vi "Experiment03.vi"() -> ()   [LabVIEW 2009]
uses:
  <vilib>/imath/engines/lvmath2/RunTimeEngine/ErrorHandling/NIMS_Finalize Error.vi
  <vilib>/imath/engines/lvmath2/RunTimeEngine/Parser/MC_Version.vi
  <vilib>/imath/engines/lvmath2/RunTimeEngine/Managers/WorkSpace/UID Generator.vi
  <vilib>/imath/engines/lvmath/Functions/Error Handling/error.ctl
  <vilib>/imath/engines/lvmath2/RunTimeEngine/NodeEndStatement/NIMS_NodeEndStatement_Output.vi
  <instcachedir>/0/NIMS_NodeEndStatement_Output_B70DDD75627E4997AAE11E9955EDAA25.lvgen/NIMS_NodeEndStatement_Output_B70DDD75627E4997AAE11E9955EDAA25_000.vi
  <vilib>/imath/engines/lvmath2/RunTimeEngine/Managers/SymbolTable/Clear UID.vi
  <vilib>/imath/engines/lvmath/Functions/Error Handling/MergeErrorsWrapper.vi
  <vilib>/imath/engines/lvmath2/RunTimeEngine/VariableToken/NIMS_VariableToken_CondDefined.vi
  <instcachedir>/0/NIMS_VariableToken_CondDefined_5641E79000FB4D628475532441475385.lvgen/NIMS_VariableToken_CondDefined_5641E79000FB4D628475532441475385_001.vi
  <vilib>/imath/engines/lvmath/Functions/Error Handling/MC_Mask_Errors.vi
  <vilib>/imath/engines/lvmath2/RunTimeEngine/BuiltInFunctions/rem/NIMS_rem_no checks.vi
  <instcachedir>/0/NIMS_rem_no checks_4CC9B305AB7E42EF90AFC4973FB32F8D.lvgen/NIMS_rem_no checks_4CC9B305AB7E42EF90AFC4973FB32F8D_000.vi
  <vilib>/imath/engines/lvmath2/RunTimeEngine/BuiltInFunctions/uint32/NIMS_uint32(real).vi
  <instcachedir>/0/NIMS_uint32(real)_FDC83D68D45943DDB8F3F934FF8A712F.lvgen/NIMS_uint32(real)_FDC83D68D45943DDB8F3F934FF8A712F_000.vi
  <vilib>/imath/engines/lvmath2/RunTimeEngine/BuiltInFunctions/double/NIMS_double.vi
  <instcachedir>/0/NIMS_double_2CE444F3CE4146B199A482FE12545E45.lvgen/NIMS_double_2CE444F3CE4146B199A482FE12545E45_000.vi
  <vilib>/imath/engines/lvmath2/RunTimeEngine/RangeToken/NIMS_Range.vi
  <instcachedir>/0/NIMS_Range_6D647EC16A744C98B5DE1D649A2D648D.lvgen/NIMS_Range_6D647EC16A744C98B5DE1D649A2D648D_001.vi
  <vilib>/imath/engines/lvmath2/RunTimeEngine/BuiltInFunctions/length/NIMS_length(GV).vi
  <instcachedir>/0/NIMS_length(GV)_7D6E94E728E145E68721C53861296D96.lvgen/NIMS_length(GV)_7D6E94E728E145E68721C53861296D96_000.vi
  <instcachedir>/0/NIMS_Range_6D647EC16A744C98B5DE1D649A2D648D.lvgen/NIMS_Range_6D647EC16A744C98B5DE1D649A2D648D_000.vi
  <vilib>/imathl/engines/lvmath/Functions/Error Handling/Create Error.vi
  <vilib>/imath/engines/lvmath2/RunTimeEngine/ReplaceToken/NIMS_Replace - V(S)=S.vi
  <instcachedir>/0/NIMS_Replace - V(S)=S_670A9E0533664C1D848C8E58B3321B6A.lvgen/NIMS_Replace - V(S)=S_670A9E0533664C1D848C8E58B3321B6A_002.vi
  <vilib>/imath/engines/lvmath2/RunTimeEngine/ReplaceToken/NIMS_Replace - Size Check _(_)=S.vi
  <instcachedir>/0/NIMS_Replace - Size Check _(_)=S_8596181D73404097BAB9CBB006194BB0.lvgen/NIMS_Replace - Size Check _(_)=S_8596181D73404097BAB9CBB006194BB0_002.vi
  <vilib>/imath/engines/lvmath2/RunTimeEngine/ReplaceToken/NIMS_Replace - Check Linear.vi
  <instcachedir>/0/NIMS_Replace - Check Linear_9243CBB174894FF6977027453DA6955E.lvgen/NIMS_Replace - Check Linear_9243CBB174894FF6977027453DA6955E_002.vi
  <vilib>/imath/engines/lvmath2/RunTimeEngine/VariableToken/NIMS_VariableToken_CondDefinedDefinedByReplace.vi
  <instcachedir>/0/NIMS_VariableToken_CondDefinedDefinedByReplace_D162CFFC24174562A9FEA619A91E1A56.lvgen/NIMS_VariableToken_CondDefinedDefinedByReplace_D162CFFC24174562A9FEA619A91E1A56_002.vi
  <vilib>/imath/engines/lvmath2/RunTimeEngine/CommandStatement/MC_CommandStatement_break.vi
  <vilib>/imath/engines/lvmath2/RunTimeEngine/LocalVariableDefStatement/MC_LocalVariableDefStatement_Display.vi
  <vilib>/imath/engines/lvmath2/RunTimeEngine/RunTimeType/NIMS_RunTimeType_From StrictType (excl LVString).vi
  <vilib>/imath/engines/lvmath2/RunTimeEngine/ArithmeticOperatorToken/NIMS_ArithmeticOperator_times.vi
  <instcachedir>/0/NIMS_ArithmeticOperator_times_3987BC660D7947CD8628C10658A43225.lvgen/NIMS_ArithmeticOperator_times_3987BC660D7947CD8628C10658A43225_001.vi
  <instcachedir>/0/NIMS_NodeEndStatement_Output_B70DDD75627E4997AAE11E9955EDAA25.lvgen/NIMS_NodeEndStatement_Output_B70DDD75627E4997AAE11E9955EDAA25_001.vi
  <instcachedir>/0/NIMS_ArithmeticOperator_times_3987BC660D7947CD8628C10658A43225.lvgen/NIMS_ArithmeticOperator_times_3987BC660D7947CD8628C10658A43225_000.vi
  <vilib>/imath/engines/lvmath2/RunTimeEngine/VariableToken/Read/NIMS_Get Elements - RV(_) - Check.vi
  <instcachedir>/0/NIMS_Get Elements - RV(_) - Check_60F12861D0564803969A5D0D0D1716CD.lvgen/NIMS_Get Elements - RV(_) - Check_60F12861D0564803969A5D0D0D1716CD_000.vi
  <instcachedir>/0/NIMS_NodeEndStatement_Output_B70DDD75627E4997AAE11E9955EDAA25.lvgen/NIMS_NodeEndStatement_Output_B70DDD75627E4997AAE11E9955EDAA25_003.vi
  <instcachedir>/0/NIMS_VariableToken_CondDefined_5641E79000FB4D628475532441475385.lvgen/NIMS_VariableToken_CondDefined_5641E79000FB4D628475532441475385_000.vi
  <instcachedir>/0/NIMS_Replace - V(S)=S_670A9E0533664C1D848C8E58B3321B6A.lvgen/NIMS_Replace - V(S)=S_670A9E0533664C1D848C8E58B3321B6A_001.vi
  <instcachedir>/0/NIMS_Replace - Size Check _(_)=S_8596181D73404097BAB9CBB006194BB0.lvgen/NIMS_Replace - Size Check _(_)=S_8596181D73404097BAB9CBB006194BB0_001.vi
  <instcachedir>/0/NIMS_Replace - Check Linear_9243CBB174894FF6977027453DA6955E.lvgen/NIMS_Replace - Check Linear_9243CBB174894FF6977027453DA6955E_001.vi
  <instcachedir>/0/NIMS_VariableToken_CondDefinedDefinedByReplace_D162CFFC24174562A9FEA619A91E1A56.lvgen/NIMS_VariableToken_CondDefinedDefinedByReplace_D162CFFC24174562A9FEA619A91E1A56_001.vi
  <vilib>/imath/engines/lvmath2/RunTimeEngine/BuiltInFunctions/abs/NIMS_abs(signed).vi
  <instcachedir>/0/NIMS_abs(signed)_C4FCB8E6058B49B797C7C8D53CA5F6EC.lvgen/NIMS_abs(signed)_C4FCB8E6058B49B797C7C8D53CA5F6EC_000.vi
  <instcachedir>/0/NIMS_NodeEndStatement_Output_B70DDD75627E4997AAE11E9955EDAA25.lvgen/NIMS_NodeEndStatement_Output_B70DDD75627E4997AAE11E9955EDAA25_002.vi
  <vilib>/imath/engines/lvmath2/RunTimeEngine/Managers/SymbolTable/NIMS_WorkSpace.lvlib
panel:
  out "Current VI path 12":string
  out "New Path for Picture 12":string
  out "Part Stripped 12":string
  out "Stripped Path 12":string
  out "Current VI path 11":string
  out "New Path for Picture 11":string
  out "Part Stripped 11":string
  out "Stripped Path 11":string
  out "Current VI path 10":string
  out "New Path for Picture 10":string
  out "Part Stripped 10":string
  out "Stripped Path 10":string
  out "Current VI path 9":string
  out "New Path for Picture 9":string
  out "Part Stripped 9":string
  out "Stripped Path 9":string
  out "Current VI path 8":string
  out "New Path for Picture 8":string
  out "Part Stripped 8":string
  out "Stripped Path 8":string
  out "Current VI path 7":string
  out "New Path for Picture 7":string
  out "Part Stripped 7":string
  out "Stripped Path 7":string
  out "Current VI path 6":string
  out "New Path for Picture 6":string
  out "Part Stripped 6":string
  out "Stripped Path 6":string
  out "Current VI path 5":string
  out "New Path for Picture 5":string
  out "Part Stripped 5":string
  out "Stripped Path 5":string
  out "Current VI path 4":string
  out "New Path for Picture 4":string
  out "Part Stripped 4":string
  out "Stripped Path 4":string
  out "Current VI path 3":string
  out "New Path for Picture 3":string
  out "Part Stripped 3":string
  out "Stripped Path 3":string
  out "Current VI path 2":string
  out "New Path for Picture 2":string
  out "Part Stripped 2":string
  out "Stripped Path 2":string
  out "Current VI path":string
  out "New Path for Picture":string
  out "Part Stripped":string
  out "Stripped Path":string
  in  "?":T1(tab)
  in  "?":dbl(slide) scale=0.1..0.5
  in  "?":enum32{"IMPEDANCE OF HORN ANTENNA"}(tab)
  in  "Reactance of Horn":dbl(slide) scale=0.0..500.0
  in  "Resistance of Horn":dbl(slide) scale=0.0..500.0
  in  "?":enum32{"SLOTTED LINE"}(tab)
  out "?":dbl[](graph)
  out "Characteristic Impedance":dbl
  in  "Slide":dbl(slide) scale=0.0..0.4
  out "Voltage 2":dbl
  out "Distance(Meter)":dbl
  in  "First Freespace Minima":bool
  in  "Second Freespace Minima":bool
  in  "First Wave-guideMinima":bool
  out "?":dbl
  out "?":dbl
  out "?":dbl
  in  "Second Wave-guide Minima":bool
  out "?":dbl
  out "?":errorcluster
  out "?":dbl
  in  "Width of the Wave-guide":bool
  in  "HELP FOR SLOTTED LINE":bool
  out "error out":errorcluster
  in  "?":enum32{"ATTENUATOR"}(tab)
  out "?":dbl[](graph)
  out "?":errorcluster
  in  "Set the value of attenuation in dB":dbl(slide) scale=0.0..100.0
  in  "HELP FOR ATTENUATOR":bool
  out "error out":errorcluster
  in  "?":enum32{"ISOLATOR"}(tab)
  out "?":dbl[](graph)
  out "?":errorcluster
  in  "?":bool
  in  "HELP FOR ISOLATOR":bool
  out "error out":errorcluster
  in  "?":enum32{"MODULATOR"}(tab)
  out "?":dbl[](graph)
  out "?":errorcluster
  in  "Modulating Frequency(KHz)":dbl(slide) scale=0.5..1.5
  in  "HELP FOR MODULATOR":bool
  out "error out":errorcluster
  in  "?":enum32{"SOURCE"}(tab)
  out "?":dbl[](graph)
  out "?":errorcluster
  in  "Voltage 3":dbl(knob) scale=0.0..20.0 scale format="%#_10g"
  in  "Frequency of carrier wave(GHz)":dbl(slide) scale=8.0..15.0
  in  "HELP FOR SOURCE":bool
  out "error out":errorcluster
  # "Backward Direction"
  # "Forward direction"
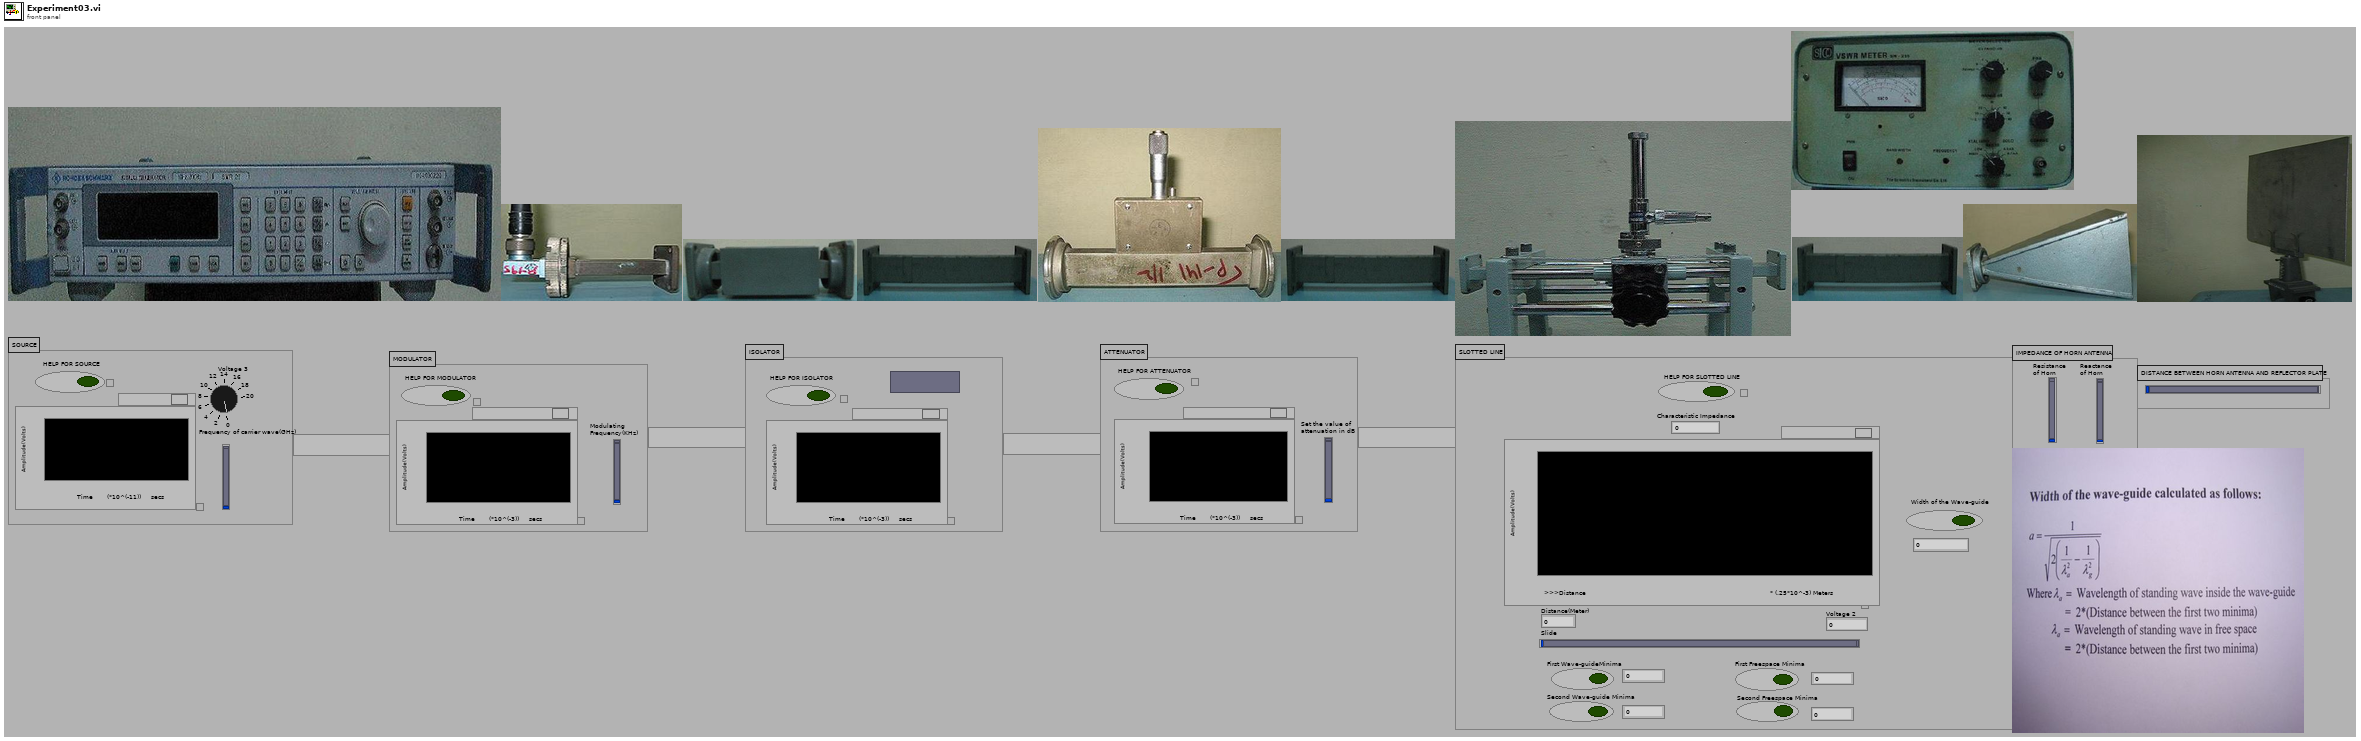
[diagram p1: front panel]
types:
  T1 = enum32{"DISTANCE BETWEEN HORN ANTENNA AND REFLECTOR PLATE"}
  T2 = typedef "imagedata.ctl" = cluster{"image type":i32, "image depth":i32, "image":u8[], "mask":u8[], "colors":u32[], "Rectangle":cluster{"left":i16, "top":i16, "right":i16, "bottom":i16}}
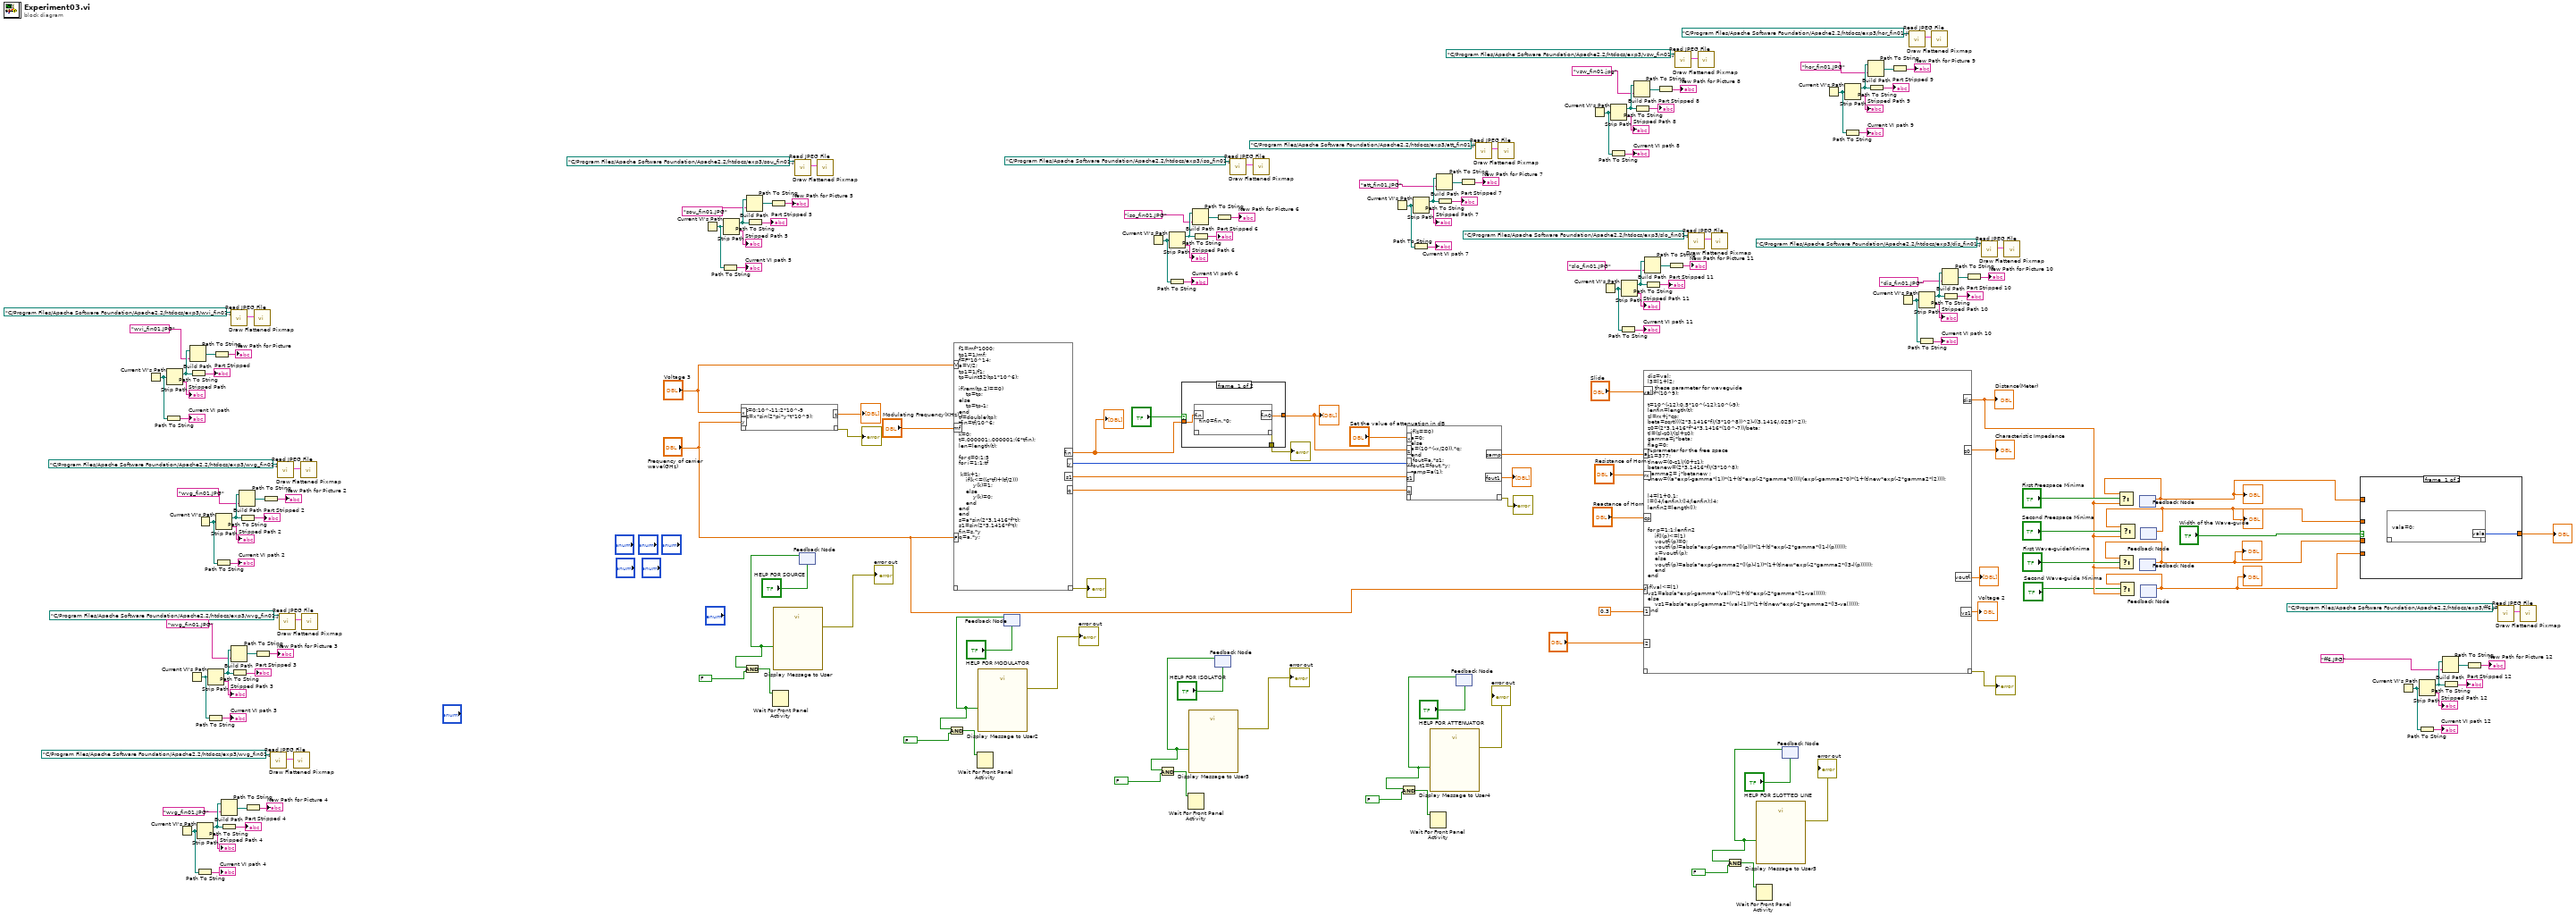
[diagram p0: block diagram]
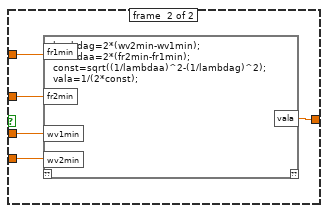
[diagram p2: hidden frame]
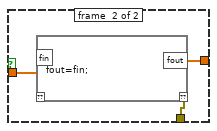
[diagram p3: hidden frame]
diagram:
  n1 = Current VI's Path() -> (path=w103:path)
  n2 = Path To String(path=w103) -> (string=→"Current VI path":string)
  n3 = Strip Path(path=w103) -> (stripped path=w108:path, name=→"Stripped Path":string)
  n4 = Current VI's Path() -> (path=w79:path)
  n5 = Current VI's Path() -> (path=w87:path)
  n6 = Build Path(base path=w108, name or relative path="wvi_fin01.JPG") -> (appended path=w101:path)
  n7 = Path To String(path=w108) -> (string=→"Part Stripped":string)
  n8 = Path To String(path=w79) -> (string=→"Current VI path 4":string)
  n9 = Current VI's Path() -> (path=w95:path)
  n10 = Strip Path(path=w79) -> (stripped path=w84:path, name=→"Stripped Path 4":string)
  n11 = Path To String(path=w87) -> (string=→"Current VI path 3":string)
  n12 = Strip Path(path=w87) -> (stripped path=w92:path, name=→"Stripped Path 3":string)
  n13 = Path To String(path=w101) -> (string=→"New Path for Picture":string)
  n14 = Path To String(path=w95) -> (string=→"Current VI path 2":string)
  n15 = Strip Path(path=w95) -> (stripped path=w100:path, name=→"Stripped Path 2":string)
  n16 = Build Path(base path=w84, name or relative path="wvg_fin01.JPG") -> (appended path=w77:path)
  n17 = Path To String(path=w84) -> (string=→"Part Stripped 4":string)
  n18 = call <vilib>:"Read JPEG File.vi"("path to JPEG file"=path "C:/Program Files/Apache Software Foundation/Apache2.2/htdocs/exp3/wvi_fin01.JPG") -> ("image data"=w117:T2)  [unwired: 1 in, 9 out]
  n19 = Build Path(base path=w92, name or relative path="wvg_fin01.JPG") -> (appended path=w85:path)
  n20 = Path To String(path=w92) -> (string=→"Part Stripped 3":string)
  n21 = Build Path(base path=w100, name or relative path="wvg_fin01.JPG") -> (appended path=w93:path)
  n22 = Path To String(path=w100) -> (string=→"Part Stripped 2":string)
  n23 = Path To String(path=w77) -> (string=→"New Path for Picture 4":string)
  n24 = call <vilib>:"Draw Flattened Pixmap.vi"("image data"=w117) -> ()  [unwired: 1 in, 8 out]
  n25 = Path To String(path=w85) -> (string=→"New Path for Picture 3":string)
  n26 = Path To String(path=w93) -> (string=→"New Path for Picture 2":string)
  n27 = call <vilib>:"Read JPEG File.vi"("path to JPEG file"=path "C:/Program Files/Apache Software Foundation/Apache2.2/htdocs/exp3/wvg_fin01.JPG") -> ("image data"=w112:T2)  [unwired: 1 in, 9 out]
  n28 = call <vilib>:"Read JPEG File.vi"("path to JPEG file"=path "C:/Program Files/Apache Software Foundation/Apache2.2/htdocs/exp3/wvg_fin01.JPG") -> ("image data"=w116:T2)  [unwired: 1 in, 9 out]
  n29 = call <vilib>:"Read JPEG File.vi"("path to JPEG file"=path "C:/Program Files/Apache Software Foundation/Apache2.2/htdocs/exp3/wvg_fin01.JPG") -> ("image data"=w114:T2)  [unwired: 1 in, 9 out]
  n30 = call <vilib>:"Draw Flattened Pixmap.vi"("image data"=w112) -> ()  [unwired: 1 in, 8 out]
  n31 = call <vilib>:"Draw Flattened Pixmap.vi"("image data"=w116) -> ()  [unwired: 1 in, 8 out]
  n32 = call <vilib>:"Draw Flattened Pixmap.vi"("image data"=w114) -> ()  [unwired: 1 in, 8 out]
  n33 = Current VI's Path() -> (path=w71:path)
  n34 = Path To String(path=w71) -> (string=→"Current VI path 5":string)
  n35 = Strip Path(path=w71) -> (stripped path=w76:path, name=→"Stripped Path 5":string)
  n36 = mathscript code="t=0:10^-11:2*10^-9\nz=x*sin(2*pi*y*t*10^9);"("x"="Voltage 3", "y"="Frequency of carrier wave(GHz)") -> ("??"=→"?":errorcluster, "z"=→"?":dbl[])  [unwired: 1 in]
  n37 = Build Path(base path=w76, name or relative path="sou_fin01.JPG") -> (appended path=w69:path)
  n38 = Path To String(path=w76) -> (string=→"Part Stripped 5":string)
  n39 = Path To String(path=w69) -> (string=→"New Path for Picture 5":string)
  n40 = call <vilib>:"Read JPEG File.vi"("path to JPEG file"=path "C:/Program Files/Apache Software Foundation/Apache2.2/htdocs/exp3/sou_fin01.JPG") -> ("image data"=w119:T2)  [unwired: 1 in, 9 out]
  n41 = feedback #1("HELP FOR SOURCE") -> (w187:bool)
  n42 = And(x=w187, y=FALSE) -> (x .and. y?=w185:bool)
  n43 = Wait For Front Panel Activity(3:w185) -> ()  [unwired: 3 out]
  n44 = call "Display Message to User"("Enable"=w187) -> ("error out"=→"error out":errorcluster, "CLOSE"=w189:bool)  [unwired: 2 in, 7 out]
  n45 = call <vilib>:"Draw Flattened Pixmap.vi"("image data"=w119) -> ()  [unwired: 1 in, 8 out]
  n46 = mathscript code="f1=mf*1000;\ntp1=1/mf;\nf=F*10^14;\na=V/2;\ntp1=1/f1;\ntp=uint32(tp1*10^6);\n\nif(rem(tp,2)==0)\n    tp=tp;\nelse\n    tp=tp-1;\nend\ntf=double(tp);\ntfin=tf/10^6;\n\nk=0;\nt=.000001:.000001:(6*tfin);\nlen=length(t);\n\nfor c=0:1:5\nfor i=1:1:tf\n  \n k=k+1;\n    if(k<=((c*tf)+(tf/2)))\n        y(k)=1;\n    else\n        y(k)=0;\n    end\nend\nend\ns=a*sin(2*3.1416*f*t);\ns1=sin(2*3.1416*f*t);\nfin=s.*y\nq=a.*y;"("V"="Voltage 3", "mf"="Modulating Frequency(KHz)", "F"="Frequency of carrier wave(GHz)") -> ("??"=→"?":errorcluster, "fin"=w155:dbl[], "y"=w152:i32[], "s1"=w151:dbl[], "q"=w150:dbl[])  [unwired: 1 in]
  "?" <- w155
  n47 = feedback #2("HELP FOR MODULATOR") -> (w181:bool)
  n48 = And(x=w181, y=FALSE) -> (x .and. y?=w179:bool)
  n49 = Wait For Front Panel Activity(3:w179) -> ()  [unwired: 3 out]
  n50 = call "Display Message to User2"("Enable"=w181) -> ("error out"=→"error out":errorcluster, "CLOSE"=w183:bool)  [unwired: 2 in, 7 out]
  n51 = Current VI's Path() -> (path=w63:path)
  n52 = Path To String(path=w63) -> (string=→"Current VI path 6":string)
  n53 = Strip Path(path=w63) -> (stripped path=w68:path, name=→"Stripped Path 6":string)
  n54 = case shown="False" "?" {
    tunnel: [w193 w214] -> w121
    tunnel: w155 -> [w194 w215]
    tunnel: [w192 w213] -> w120
    frame #0 {
      n55 = mathscript code="fin0=fin.*0;"("fin"=w194) -> ("??"=w192:errorcluster, "fin0"=w193:dbl[])  [unwired: 1 in]
    }
    frame #1 {
      n56 = mathscript code="fout=fin;"("fin"=w215) -> ("??"=w213:errorcluster, "fout"=w214:dbl[])  [unwired: 1 in]
    }
  }
  "?" <- w121
  "?" <- w120
  n57 = Build Path(base path=w68, name or relative path="iso_fin01.JPG") -> (appended path=w61:path)
  n58 = Path To String(path=w68) -> (string=→"Part Stripped 6":string)
  n59 = feedback #3("HELP FOR ISOLATOR") -> (w175:bool)
  n60 = And(x=w175, y=FALSE) -> (x .and. y?=w173:bool)
  n61 = Wait For Front Panel Activity(3:w173) -> ()  [unwired: 3 out]
  n62 = call "Display Message to User3"("Enable"=w175) -> ("error out"=→"error out":errorcluster, "CLOSE"=w177:bool)  [unwired: 2 in, 7 out]
  n63 = Path To String(path=w61) -> (string=→"New Path for Picture 6":string)
  n64 = call <vilib>:"Read JPEG File.vi"("path to JPEG file"=path "C:/Program Files/Apache Software Foundation/Apache2.2/htdocs/exp3/iso_fin01.JPG") -> ("image data"=w118:T2)  [unwired: 1 in, 9 out]
  n65 = call <vilib>:"Draw Flattened Pixmap.vi"("image data"=w118) -> ()  [unwired: 1 in, 8 out]
  n66 = Current VI's Path() -> (path=w55:path)
  n67 = mathscript code="if(z==0)\na=0; \nelse\na=(10^(-x/20)).*q;\nend\n fout=a.*s1;\nfout1=fout.*y;\nsamp=a(1);"("x"="Set the value of attenuation in dB", "z"=w121, "y"=w152, "s1"=w151, "q"=w150) -> ("??"=→"?":errorcluster, "samp"=w146:dbl, "fout1"=→"?":dbl[])  [unwired: 1 in]
  n68 = Path To String(path=w55) -> (string=→"Current VI path 7":string)
  n69 = Strip Path(path=w55) -> (stripped path=w60:path, name=→"Stripped Path 7":string)
  n70 = Build Path(base path=w60, name or relative path="att_fin01.JPG") -> (appended path=w53:path)
  n71 = Path To String(path=w60) -> (string=→"Part Stripped 7":string)
  n72 = feedback #4("HELP FOR ATTENUATOR") -> (w169:bool)
  n73 = And(x=w169, y=FALSE) -> (x .and. y?=w167:bool)
  n74 = Wait For Front Panel Activity(3:w167) -> ()  [unwired: 3 out]
  n75 = call "Display Message to User4"("Enable"=w169) -> ("error out"=→"error out":errorcluster, "CLOSE"=w171:bool)  [unwired: 2 in, 7 out]
  n76 = Path To String(path=w53) -> (string=→"New Path for Picture 7":string)
  n77 = call <vilib>:"Read JPEG File.vi"("path to JPEG file"=path "C:/Program Files/Apache Software Foundation/Apache2.2/htdocs/exp3/att_fin01.JPG") -> ("image data"=w115:T2)  [unwired: 1 in, 9 out]
  n78 = call <vilib>:"Draw Flattened Pixmap.vi"("image data"=w115) -> ()  [unwired: 1 in, 8 out]
  n79 = Current VI's Path() -> (path=w47:path)
  n80 = Current VI's Path() -> (path=w23:path)
  n81 = Path To String(path=w47) -> (string=→"Current VI path 8":string)
  n82 = Strip Path(path=w47) -> (stripped path=w52:path, name=→"Stripped Path 8":string)
  n83 = Path To String(path=w23) -> (string=→"Current VI path 11":string)
  n84 = Strip Path(path=w23) -> (stripped path=w28:path, name=→"Stripped Path 11":string)
  n85 = Build Path(base path=w52, name or relative path="vsw_fin01.jpg") -> (appended path=w45:path)
  n86 = Path To String(path=w52) -> (string=→"Part Stripped 8":string)
  n87 = mathscript code="dis=val;\nl3=l1+l2;\n% these parameter for waveguide\nf=f*(10^9);\n\nt=10^(-12):0.5*10^(-12):10^(-9);\nlenfin=length(t);\nzl=rx+j*cp;\nbeta=sqrt((((2*3.1416*f)/(3*10^8))^2)-((3.1416/.025)^2));\nz0=(2*3.1416*f*4*3.1416*(10^-7))/beta;\ntl=(zl-z0)/(zl+z0);\ngamma=j*beta;\nflag=0;\n%prameter for the free space\nz1=377;\ntlnew=(0-z1)/(0+z1);\nbetanew=(2*3.1416*f)/(3*10^8);\ngamma2= j*betanew ;\nanew=((a*exp(-gamma*l1))*(1+(tl*exp(-2*gamma*0))))/(exp(-gamma2*0)*(1+(tlnew*exp(-2*gamma2*l2))));\n\n\nl4=l1+0.1;\nl=(l4/lenfin):(l4/lenfin):l4;\nlenfin2=length(l);\n\n\n\nfor p=1:1:lenfin2\n    if(l(p)<=l1)\n    voutfi(p)=0;\n    voutfi(p)=abs(a*exp(-gamma*(l(p)))*(1+(tl*exp(-2*gamma*(l1-l(p))))));\n    x=voutfi(p);\n    else\n    voutfi(p)=abs(a*exp(-gamma2*(l(p)-l1))*(1+(tlnew*exp(-2*gamma2*(l3-l(p))))));\n    end\nend\n\nif(val<=l1)\nvs1=abs(a*exp(-gamma*(val))*(1+(tl*exp(-2*gamma*(l1-val)))));\nelse\n    vs1=abs(a*exp(-gamma2*(val-l1))*(1+(tlnew*exp(-2*gamma2*(l3-val)))));\nend"("val"="Slide", "a"=w146, "rx"="Resistance of Horn", "cp"="Reactance of Horn", "f"="Frequency of carrier wave(GHz)", "l1"=0.3 ("Real"), "l2"="?") -> ("??"=→"?":errorcluster, "dis"=w124:dbl, "z0"=→"Characteristic Impedance":cdb, "voutfi"=→"?":dbl[], "vs1"=→"Voltage 2":dbl)  [unwired: 1 in]
  "Distance(Meter)" <- w124
  n88 = Build Path(base path=w28, name or relative path="slo_fin01.JPG") -> (appended path=w21:path)
  n89 = Path To String(path=w28) -> (string=→"Part Stripped 11":string)
  n90 = Path To String(path=w45) -> (string=→"New Path for Picture 8":string)
  n91 = Path To String(path=w21) -> (string=→"New Path for Picture 11":string)
  n92 = call <vilib>:"Read JPEG File.vi"("path to JPEG file"=path "C:/Program Files/Apache Software Foundation/Apache2.2/htdocs/exp3/vsw_fin01.JPG") -> ("image data"=w109:T2)  [unwired: 1 in, 9 out]
  n93 = call <vilib>:"Read JPEG File.vi"("path to JPEG file"=path "C:/Program Files/Apache Software Foundation/Apache2.2/htdocs/exp3/slo_fin01.JPG") -> ("image data"=w113:T2)  [unwired: 1 in, 9 out]
  n94 = call <vilib>:"Draw Flattened Pixmap.vi"("image data"=w109) -> ()  [unwired: 1 in, 8 out]
  n95 = call <vilib>:"Draw Flattened Pixmap.vi"("image data"=w113) -> ()  [unwired: 1 in, 8 out]
  n96 = feedback #5("HELP FOR SLOTTED LINE") -> (w163:bool)
  n97 = And(x=w163, y=FALSE) -> (x .and. y?=w161:bool)
  n98 = Wait For Front Panel Activity(3:w161) -> ()  [unwired: 3 out]
  n99 = call "Display Message to User5"("Enable"=w163) -> ("error out"=→"error out":errorcluster, "CLOSE"=w165:bool)  [unwired: 2 in, 7 out]
  n100 = Current VI's Path() -> (path=w39:path)
  n101 = Path To String(path=w39) -> (string=→"Current VI path 9":string)
  n102 = Strip Path(path=w39) -> (stripped path=w44:path, name=→"Stripped Path 9":string)
  n103 = Build Path(base path=w44, name or relative path="hor_fin01.JPG") -> (appended path=w37:path)
  n104 = Path To String(path=w44) -> (string=→"Part Stripped 9":string)
  n105 = Path To String(path=w37) -> (string=→"New Path for Picture 9":string)
  n106 = Current VI's Path() -> (path=w31:path)
  n107 = call <vilib>:"Read JPEG File.vi"("path to JPEG file"=path "C:/Program Files/Apache Software Foundation/Apache2.2/htdocs/exp3/hor_fin01.JPG") -> ("image data"=w111:T2)  [unwired: 1 in, 9 out]
  n108 = Path To String(path=w31) -> (string=→"Current VI path 10":string)
  n109 = Strip Path(path=w31) -> (stripped path=w36:path, name=→"Stripped Path 10":string)
  n110 = call <vilib>:"Draw Flattened Pixmap.vi"("image data"=w111) -> ()  [unwired: 1 in, 8 out]
  n111 = Build Path(base path=w36, name or relative path="dis_fin01.JPG") -> (appended path=w29:path)
  n112 = Path To String(path=w36) -> (string=→"Part Stripped 10":string)
  n113 = Path To String(path=w29) -> (string=→"New Path for Picture 10":string)
  n114 = call <vilib>:"Read JPEG File.vi"("path to JPEG file"=path "C:/Program Files/Apache Software Foundation/Apache2.2/htdocs/exp3/dis_fin01.JPG") -> ("image data"=w110:T2)  [unwired: 1 in, 9 out]
  n115 = call <vilib>:"Draw Flattened Pixmap.vi"("image data"=w110) -> ()  [unwired: 1 in, 8 out]
  n116 = feedback #6() -> (w132:dbl)  [unwired: 1 in]
  "?" <- w132
  n117 = Select(t=w132, s="First Freespace Minima", f=w124) -> (s? t:f=w134:dbl)
  n118 = feedback #7() -> (w126:dbl)  [unwired: 1 in]
  "?" <- w126
  n119 = Select(t=w126, s="First Wave-guideMinima", f=w124) -> (s? t:f=w128:dbl)
  n120 = feedback #8() -> (w122:dbl)  [unwired: 1 in]
  "?" <- w122
  n121 = Select(t=w122, s="Second Wave-guide Minima", f=w124) -> (s? t:f=w125:dbl)
  n122 = feedback #9() -> (w129:dbl)  [unwired: 1 in]
  "?" <- w129
  n123 = Select(t=w129, s="Second Freespace Minima", f=w124) -> (s? t:f=w131:dbl)
  n124 = case shown="True" "Width of the Wave-guide" {
    tunnel: [w232 w247] -> w136
    tunnel: w132 -> [_ w251]
    tunnel: w129 -> [_ w250]
    tunnel: w126 -> [_ w249]
    tunnel: w122 -> [_ w248]
    frame #0 {
      n125 = mathscript code="vala=0;"() -> ("vala"=w232:i32)  [unwired: 1 in, 1 out]
    }
    frame #1 {
      n126 = mathscript code="lambdag=2*(wv2min-wv1min);\nlambdaa=2*(fr2min-fr1min);\nconst=sqrt((1/lambdaa)^2-(1/lambdag)^2);\nvala=1/(2*const);"("fr1min"=w251, "fr2min"=w250, "wv1min"=w249, "wv2min"=w248) -> ("vala"=w247:cdb)  [unwired: 1 in, 1 out]
    }
  }
  "?" <- w136
  n127 = Current VI's Path() -> (path=w15:path)
  n128 = Path To String(path=w15) -> (string=→"Current VI path 12":string)
  n129 = Strip Path(path=w15) -> (stripped path=w20:path, name=→"Stripped Path 12":string)
  n130 = Build Path(base path=w20, name or relative path="ff6.JPG") -> (appended path=w13:path)
  n131 = Path To String(path=w20) -> (string=→"Part Stripped 12":string)
  n132 = Path To String(path=w13) -> (string=→"New Path for Picture 12":string)
  n133 = call <vilib>:"Read JPEG File.vi"("path to JPEG file"=path "C:/Program Files/Apache Software Foundation/Apache2.2/htdocs/exp3/ff6.JPG") -> ("image data"=w160:T2)  [unwired: 1 in, 9 out]
  n134 = call <vilib>:"Draw Flattened Pixmap.vi"("image data"=w160) -> ()  [unwired: 1 in, 8 out]
